vi "Teleop.vi"(10 "Match Info":T1={"Autonomous Elapsed Seconds"=0.0, "TeleOp Elapsed Seconds"=0.0, "Disabled Elapsed Seconds"=0.0, "Visited Autonomous"=FALSE, "Visited TeleOp"=FALSE, "Visited Disabled"=FALSE, "Autonomous Settings"={"Autonomous Style"=enum."Independent", "VI Refnum"=refnum}}, 11 "Call Context":T2) -> ()   [LabVIEW 2014]
doc: "This VI is called for each TeleOp packet received from the DS where the robot is not disabled. It is often used to read from the joysticks and update I/O or to update setpoints for timed control loops. It should complete and return within 20 milliseconds or it may miss DS packets."
uses:
  <vilib>/Rock Robotics/WPI/DriverStation/WPI_DriverStationDerivedRobotMode.ctl
  <vilib>/Rock Robotics/WPI/DriverStation/WPI_DriverStationMatch Info.ctl
  <vilib>/Rock Robotics/Network Tables/SD Read Boolean.vi
  <vilib>/Rock Robotics/Network Tables/SD Read Number.vi
  <vilib>/Rock Robotics/WPI/RobotDrive/WPI_RobotDriveGetSetRefNum.vi
  <vilib>/Rock Robotics/WPI/Joystick/WPI_JoystickGetSetRefNum.vi
  <vilib>/Rock Robotics/Network Tables/SD Write Numeric Array.vi
  <vilib>/Rock Robotics/Network Tables/SD Write Boolean Array.vi
  <vilib>/Rock Robotics/WPI/RobotDrive/WPI_RobotDriveMecanumDrive_Cartesian.vi
  Robot Global Data.vi
  <vilib>/addons/control/pid/NI_PID_pid.lvlib
  <vilib>/addons/control/pid/pid.llb/PID (DBL).vi
panel:
  out "Sample Slider 0":dbl(slide) scale=0.0..5.0
  out "Sample Boolean 1":bool
  out "Sample Boolean 0":bool
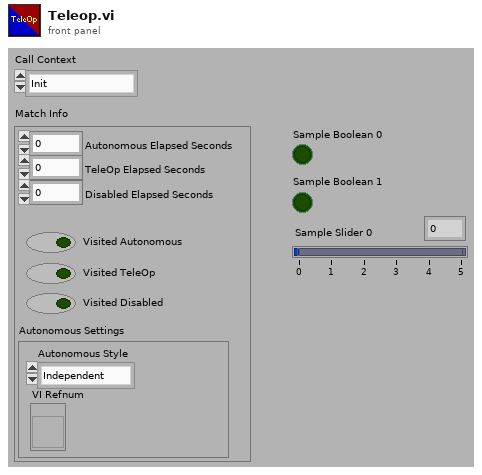
[diagram p1: front panel]
types:
  T1 = typedef "WPI_DriverStationMatch Info.ctl" = cluster{"Autonomous Elapsed Seconds":dbl, "TeleOp Elapsed Seconds":dbl, "Disabled Elapsed Seconds":dbl, "Visited Autonomous":bool, "Visited TeleOp":bool, "Visited Disabled":bool, "Autonomous Settings":cluster{"Autonomous Style":enum16{"Iterative", "Independent"}, "VI Refnum":refnum<vi>}}
  T2 = typedef "WPI_DriverStationDerivedRobotMode.ctl" = enum16{"Init", "Execute", "Stop"}
  T3 = enum16{"straight", "L1", "L2", "R1", "R2", "trigger"}
  T4 = typedef "WPI_JoystickDevRef.ctl" = cluster{"Device":T5}
  T5 = typedef "WPI_JoystickDeviceEnum.ctl" = enum16{"USB 0", "USB 1", "USB 2", "USB 3", "USB 4", "USB 5"}
  T6 = typedef "WPI_GyroDevRef.ctl" = cluster{"DevStatus":errorcluster, "Analog Module":T7, "Analog Channel":T8, "Offset":dbl, "Gain (VoltsPerDegree/Second)":dbl}
  T7 = typedef "FPGA_TypedefAnalogModule.ctl" = enum16{"Controller 1"}
  T8 = typedef "FPGA_AIChannel.ctl" = enum8{"AI 0", "AI 1", "AI 2", "AI 3", "AI MXP 0", "AI MXP 1", "AI MXP 2", "AI MXP 3", "Invalid"}
  T9 = typedef "WPI_RobotDriveDevRef.ctl" = cluster{"DevStatus":errorcluster, "Motors[]":T10[], "Square Inputs":bool, "Max Output":dbl}
  T10 = typedef "WPI_MotorControlDeviceRef.ctl" = cluster{"DeviceStatus":errorcluster, "Type":T11, "PWM":cluster{"Controller":T12, "PWM Channel":T13, "DeadBand":T14}, "CAN":cluster{"Device Number":u8, "Control Mode":T15, "Semaphore":T16, "Max Vout":dbl, "TalonSRX Control Mode":T17}, "Invert":bool, "TransformRef":T18, "InvTransformRef":T18}
  T11 = typedef "WPI_MotorControlType.ctl" = enum16{"PWM", "CAN", "CANTalonSRX"}
  T12 = typedef "FPGA_TypedefDigitalModule.ctl" = enum16{"Controller 1"}
  T13 = typedef "FPGA_DIOPWMChannel.ctl" = enum8{"PWM 0", "PWM 1", "PWM 2", "PWM 3", "PWM 4", "PWM 5", "PWM 6", "PWM 7", "PWM 8", "PWM 9", "PWM MXP 0", "PWM MXP 1", "PWM MXP 2", "PWM MXP 3", "PWM MXP 4", "PWM MXP 5", "PWM MXP 6", "PWM MXP 7", "PWM MXP 8", "PWM MXP 9", "Invalid"}
  T14 = typedef "WPI_PWMDeadband.ctl" = cluster{"Name":string, "maxPositivePwm":i32, "minPositivePwm":i32, "centerPwm":i32, "maxNegativePwm":i32, "minNegativePwm":i32, "angularRange":u16}
  T15 = typedef "WPI_CANJaguar_ControlMode.ctl" = enum8{"Percent VBus", "Current", "Speed", "Position", "Voltage"}
  T16 = typedef "Semaphore RefNum" = refnum<k1>
  T17 = typedef "WPI_CANTalonSRX_APIControlMode.ctl" = enum8{"Percent VBus", "Speed", "Position", "Slave", "Unchanged / Invalid"}
  T18 = typedef "WPI_PWMTransform_ConPane.ctl" = refnum<vi>
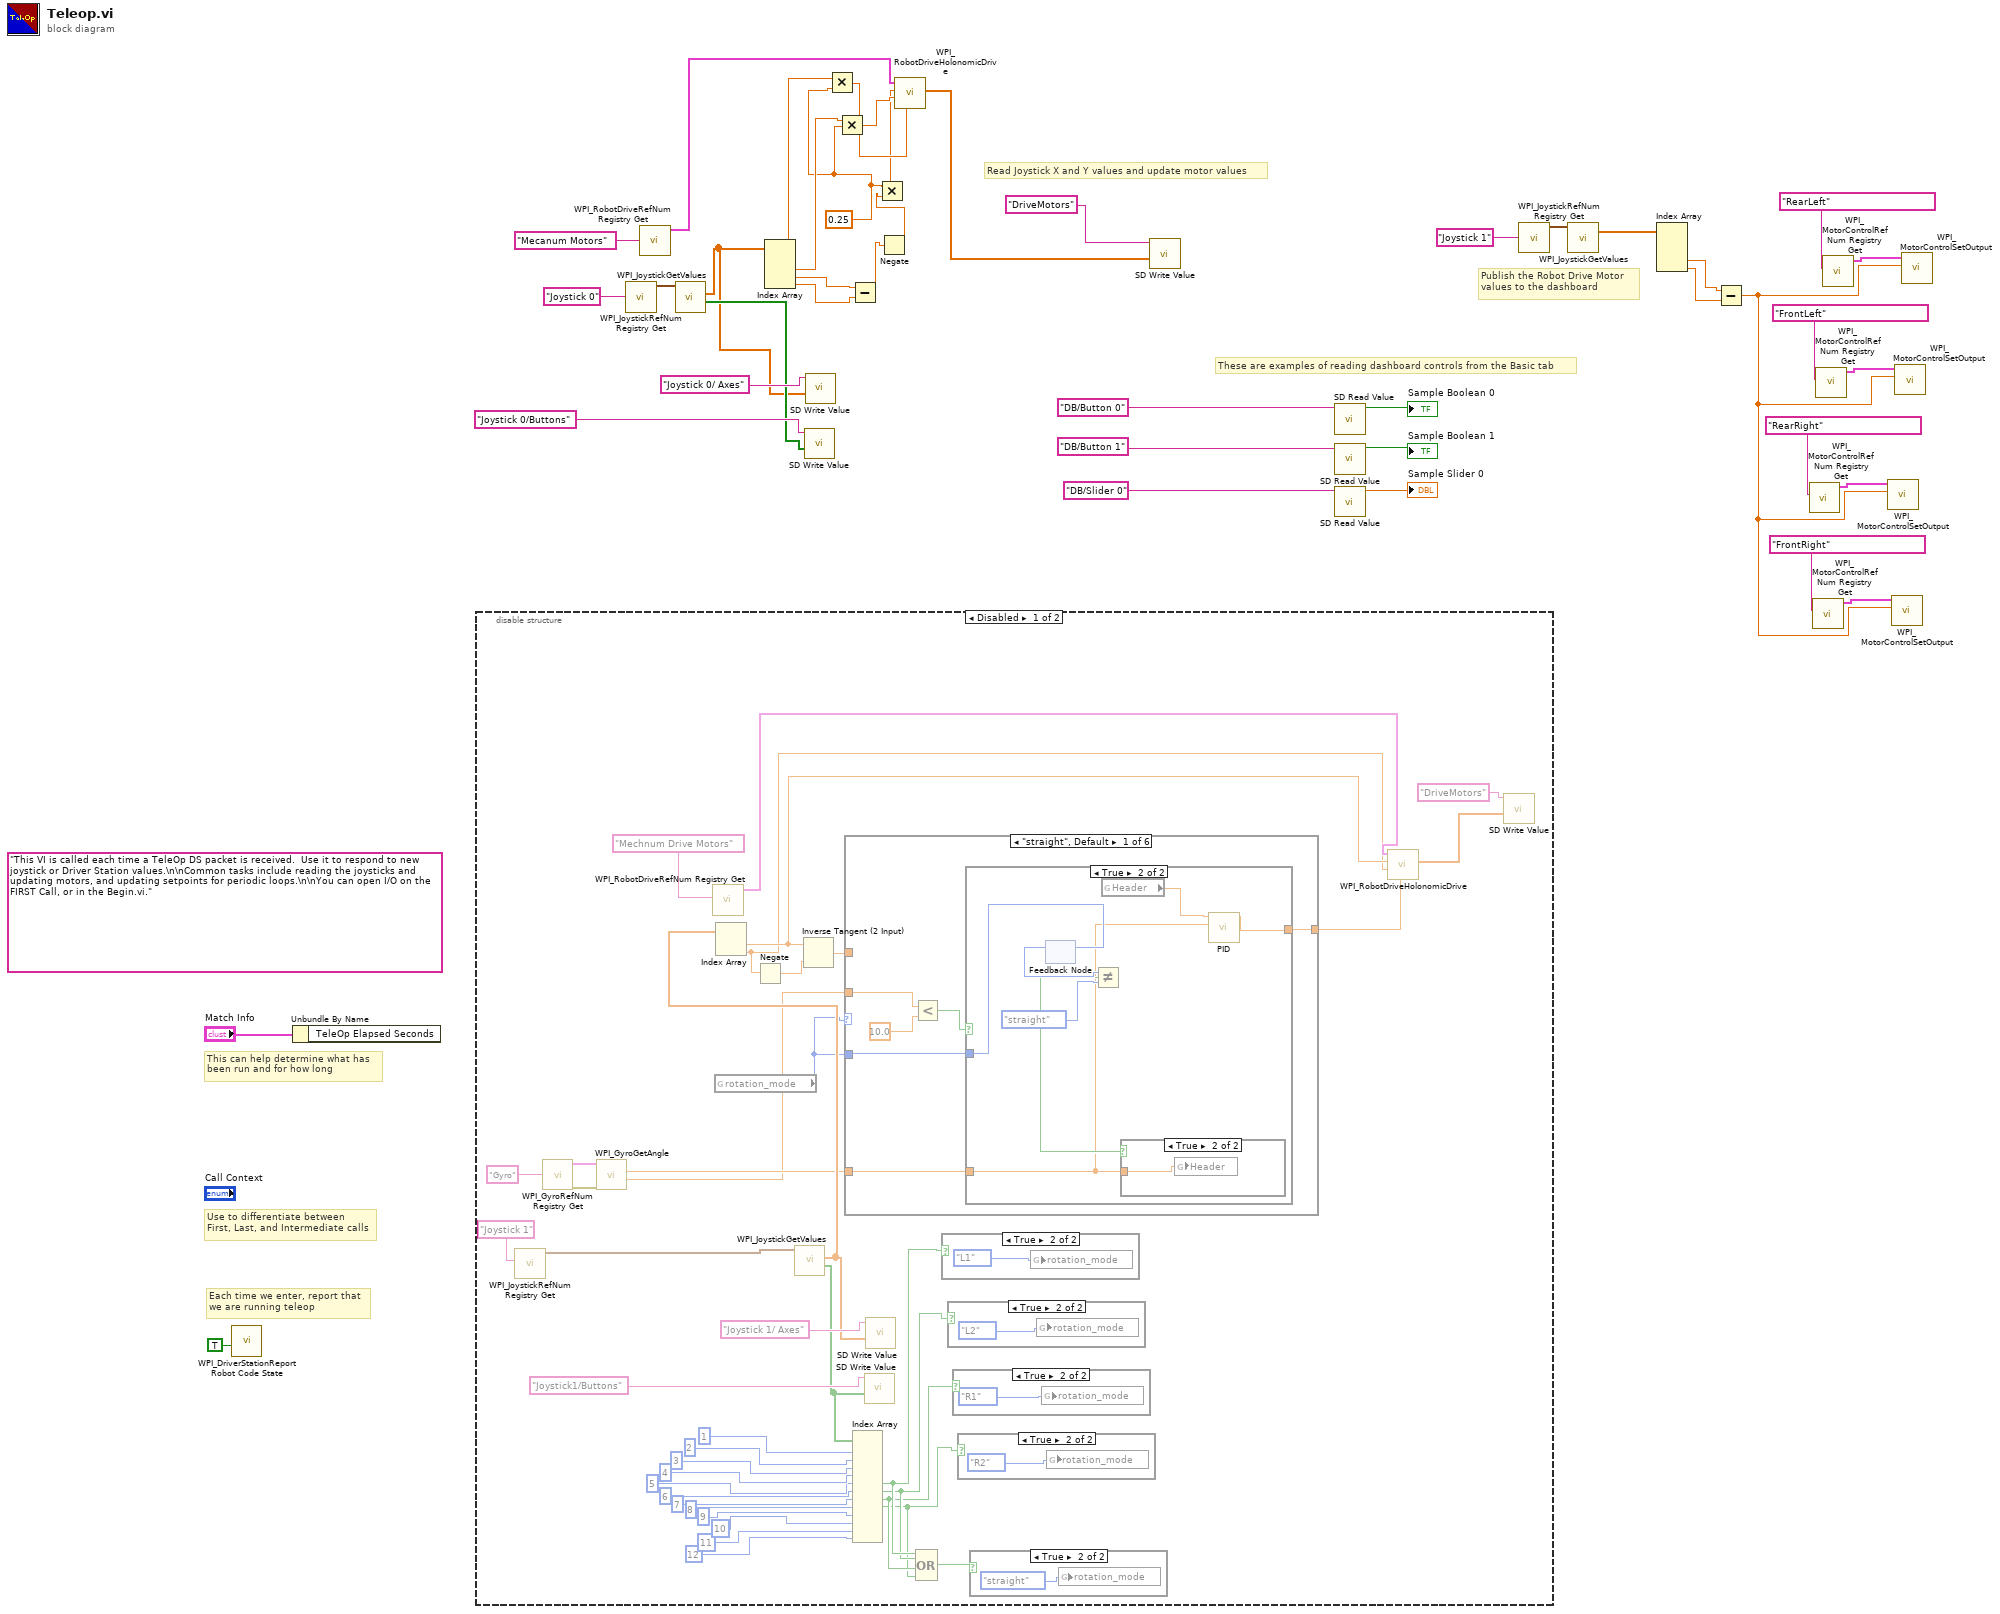
[diagram p0: block diagram]
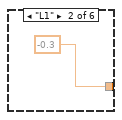
[diagram p9: hidden frame]
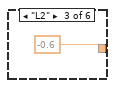
[diagram p10: hidden frame]
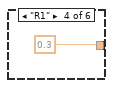
[diagram p11: hidden frame]
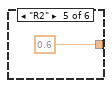
[diagram p12: hidden frame]
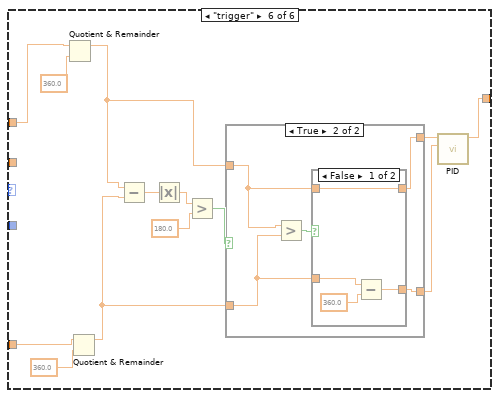
[diagram p13: hidden frame]
diagram:
  w3 = 0.25
  (unwired) "This VI is called each time a TeleOp DS packet is received.  Use it to respond to new joystick or Driver Station values.\n\nCommon tasks include reading the joysticks and updating motors, and updating setpoints for periodic loops.\n\nYou can open I/O on the FIRST Call, or in the Begin.vi."
  # "Publish the Robot Drive Motor\nvalues to the dashboard"
  # "Read Joystick X and Y values and update motor values"
  # "These are examples of reading dashboard controls from the Basic tab"
  # "Each time we enter, report that\nwe are running teleop"
  # "Use to differentiate between\nFirst, Last, and Intermediate calls"
  # "This can help determine what has\nbeen run and for how long"
  n1 = call <vilib>:"WPI_DriverStationReport Robot Code State.vi"("TeleOp"=TRUE ("Autonomous")) -> ()  [unwired: 10 in, 1 out]
  n2 = Unbundle By Name("Match Info") -> ()  [unwired: 1 out]
  n3 = disable-structure shown="Disabled" {
    frame Disabled {
      n4 = call <vilib>:"WPI_JoystickRefNum Registry Get.vi"("refnum name"="Joystick 1") -> ("JoystickDevRef"=w75:T4)  [unwired: 1 in, 9 out]
      n5 = call <vilib>:"WPI_GyroRefNum Registry Get.vi"("refnum name"="Gyro") -> ("error out"=w65:errorcluster, "GyroDevRef"=w64:T6)  [unwired: 9 in]
      n6 = call <vilib>:"WPI_GyroGetAngle.vi"("error in (no error)"=w65, "GyroDevRef"=w64) -> ("Angular Rate"=w43:dbl, "Angle"=w44:dbl)  [unwired: 6 in, 2 out]
      n7 = call <vilib>:"WPI_RobotDriveRefNum Registry Get.vi"("refnum name"="Mechnum Drive Motors") -> ("RobotDriveDevRef"=w70:T9)  [unwired: 1 in, 9 out]
      n8 = global read "Robot Global Data.vi" "rotation_mode"() -> (w51:T3)
      n9 = call <vilib>:"WPI_JoystickGetValues.vi"("JoystickDevRef"=w75) -> ("Buttons"=w74:bool[], "Axes"=w72:dbl[])  [unwired: 6 in, 3 out]
      n10 = Index Array(array=w72) -> (element #1=w71:dbl, element #2=w69:dbl)  [unwired: 2 in]
      n11 = Negate(x=w69) -> (-x=w68:dbl)
      n12 = Inverse Tangent (2 Input)(1:w68, 2:w71) -> (0:w67:dbl)
      n13 = case shown="\"straight\", Default" w51 {
        tunnel: w67 -> [_ _ _ _ _ w116]
        tunnel: w51 -> [w91 _ _ _ _ _]
        tunnel: [w86 -0.3 -0.6 0.3 0.6 w107] -> w50
        tunnel: w44 -> [w90 _ _ _ _ w114]
        tunnel: w43 -> [w87 _ _ _ _ _]
        frame "straight", Default {
          n14 = Less?(x=w87, y=10.0) -> (x < y?=w89:bool)
          n15 = case shown="True" w89 {
            tunnel: [w92 w95] -> w86
            tunnel: w91 -> [_ w94]
            tunnel: w90 -> [w92 w93]
            frame False {
            }
            frame True {
              n16 = feedback #1() -> (w99:T3)  [unwired: 1 in]
              n17 = feedback-in #1(w94) -> ()
              n18 = Not Equal?(x=w99, y=T3."straight") -> (x != y?=w97:bool)
              n19 = global read "Robot Global Data.vi" "Header"() -> (w96:dbl)
              n20 = case shown="True" w97 {
                tunnel: w93 -> [_ w100]
                frame False {
                }
                frame True {
                  n21 = global write "Robot Global Data.vi" "Header"(w100) -> ()
                }
              }
              n22 = call-poly <vilib>:"PID.vi"("process variable"=w93, "setpoint"=w96) -> ("output"=w95:dbl)  [unwired: 8 in, 1 out]
            }
          }
        }
        frame "L1" {
        }
        frame "L2" {
        }
        frame "R1" {
        }
        frame "R2" {
        }
        frame "trigger" {
          n23 = Quotient & Remainder(x=w116, y=360.0) -> (x-y*floor(x/y)=w109:dbl)  [unwired: 1 out]
          n24 = Quotient & Remainder(x=w114, y=360.0) -> (x-y*floor(x/y)=w108:dbl)  [unwired: 1 out]
          n25 = Subtract(x=w109, y=w108) -> (x-y=w113:dbl)
          n26 = Absolute Value(x=w113) -> (abs(x)=w112:dbl)
          n27 = Greater?(x=w112, y=180.0) -> (0:w110:bool)
          n28 = case shown="True" w110 {
            tunnel: w109 -> [w118 w123]
            tunnel: w108 -> [w119 w122]
            tunnel: [w119 w120] -> w106
            tunnel: [w118 w121] -> w105
            frame False {
            }
            frame True {
              n29 = Greater?(x=w123, y=w122) -> (0:w124:bool)
              n30 = case shown="False" w124 {
                tunnel: w123 -> [w127 w130]
                tunnel: w122 -> [w126 w129]
                tunnel: [w127 w130] -> w121
                tunnel: [w125 w129] -> w120
                frame False {
                  n31 = Subtract(x=w126, y=360.0) -> (x-y=w125:dbl)
                }
                frame True {
                }
              }
            }
          }
          n32 = call-poly <vilib>:"PID.vi"("process variable"=w106, "setpoint"=w105) -> ("output"=w107:dbl)  [unwired: 8 in, 1 out]
        }
      }
      n33 = Index Array(array=w74, index #1=1, index #2=2, index #3=3, index #4=4, index #5=5, index #6=6, index #7=7, index #8=8, index #9=9, index #10=10, index #11=11, index #12=12) -> (element #5=w49:bool, element #6=w48:bool, element #7=w47:bool, element #8=w46:bool)  [unwired: 8 out]
      n34 = call-poly <vilib>:"SD Write Value.vi"("Boolean Array"=w74, "Name"="Joystick1/Buttons") -> ()  [unwired: 8 in, 2 out]
      n35 = call-poly <vilib>:"SD Write Value.vi"("Numeric Array"=w72, "Name"="Joystick 1/ Axes") -> ()  [unwired: 8 in, 2 out]
      n36 = Compound Arithmetic op=OR(w49, w48, w47, w46) -> (w45:bool)
      n37 = case shown="True" w49 {
        frame False {
        }
        frame True {
          n38 = global write "Robot Global Data.vi" "rotation_mode"(T3."L1") -> ()
        }
      }
      n39 = case shown="True" w48 {
        frame False {
        }
        frame True {
          n40 = global write "Robot Global Data.vi" "rotation_mode"(T3."L2") -> ()
        }
      }
      n41 = case shown="True" w47 {
        frame False {
        }
        frame True {
          n42 = global write "Robot Global Data.vi" "rotation_mode"(T3."R1") -> ()
        }
      }
      n43 = case shown="True" w46 {
        frame False {
        }
        frame True {
          n44 = global write "Robot Global Data.vi" "rotation_mode"(T3."R2") -> ()
        }
      }
      n45 = case shown="True" w45 {
        frame False {
        }
        frame True {
          n46 = global write "Robot Global Data.vi" "rotation_mode"(T3."straight") -> ()
        }
      }
      n47 = call-poly <vilib>:"WPI_RobotDriveHolonomicDrive.vi"("Rotation"=w50, "Y"=w69, "X"=w71, "RobotDriveDevRef"=w70) -> ("Motor Values"=w77:dbl[])  [unwired: 5 in, 2 out]
      n48 = call-poly <vilib>:"SD Write Value.vi"("Numeric Array"=w77, "Name"="DriveMotors") -> ()  [unwired: 8 in, 2 out]
    }
    frame Enabled {
    }
  }
  n49 = call <vilib>:"WPI_JoystickRefNum Registry Get.vi"("refnum name"="Joystick 0") -> ("JoystickDevRef"=w23:T4)  [unwired: 9 in, 1 out]
  n50 = call <vilib>:"WPI_RobotDriveRefNum Registry Get.vi"("refnum name"="Mecanum Motors") -> ("RobotDriveDevRef"=w14:T9)  [unwired: 9 in, 1 out]
  n51 = call <vilib>:"WPI_JoystickGetValues.vi"("JoystickDevRef"=w23) -> ("Buttons"=w20:bool[], "Axes"=w19:dbl[])  [unwired: 6 in, 3 out]
  n52 = Index Array(array=w19) -> (element #1=w13:dbl, element #2=w12:dbl, element #3=w6:dbl, element #4=w5:dbl)  [unwired: 4 in]
  n53 = call-poly <vilib>:"SD Write Value.vi"("Boolean Array"=w20, "Name"="Joystick 0/Buttons") -> ()  [unwired: 8 in, 2 out]
  n54 = call-poly <vilib>:"SD Write Value.vi"("Numeric Array"=w19, "Name"="Joystick 0/ Axes") -> ()  [unwired: 8 in, 2 out]
  n55 = Multiply(x=w13, y=w3) -> (x*y=w7:dbl)
  n56 = Multiply(x=w12, y=w3) -> (x*y=w11:dbl)
  n57 = Subtract(x=w6, y=w5) -> (x-y=w4:dbl)
  n58 = Negate(x=w4) -> (-x=w2:dbl)
  n59 = Multiply(x=w3, y=w2) -> (x*y=w1:dbl)
  n60 = call-poly <vilib>:"WPI_RobotDriveHolonomicDrive.vi"("Rotation"=w7, "Y"=w11, "X"=w1, "RobotDriveDevRef"=w14) -> ("Motor Values"=w18:dbl[])  [unwired: 5 in, 2 out]
  n61 = call-poly <vilib>:"SD Write Value.vi"("Numeric Array"=w18, "Name"="DriveMotors") -> ()  [unwired: 8 in, 2 out]
  n62 = call-poly <vilib>:"SD Read Value.vi"("Name"="DB/Button 0" ("refnum name")) -> ("Boolean"=→"Sample Boolean 0":bool)  [unwired: 8 in, 2 out]
  n63 = call-poly <vilib>:"SD Read Value.vi"("Name"="DB/Button 1" ("refnum name")) -> ("Boolean"=→"Sample Boolean 1":bool)  [unwired: 8 in, 2 out]
  n64 = call-poly <vilib>:"SD Read Value.vi"("Name"="DB/Slider 0" ("refnum name")) -> ("Numeric"=→"Sample Slider 0":dbl)  [unwired: 8 in, 2 out]
  n65 = call <vilib>:"WPI_JoystickRefNum Registry Get.vi"("refnum name"="Joystick 1") -> ("JoystickDevRef"=w15:T4)  [unwired: 9 in, 1 out]
  n66 = call <vilib>:"WPI_JoystickGetValues.vi"("JoystickDevRef"=w15) -> ("Axes"=w10:dbl[])  [unwired: 6 in, 4 out]
  n67 = Index Array(array=w10) -> (element #3=w9:dbl, element #4=w8:dbl)  [unwired: 4 in, 2 out]
  n68 = Subtract(x=w9, y=w8) -> (x-y=w26:dbl)
  n69 = call <vilib>:"WPI_MotorControlRefNum Registry Get.vi"("refnum name"="RearRight") -> ("MotorControlDevRef"=w28:T10)  [unwired: 9 in, 1 out]
  n70 = call <vilib>:"WPI_MotorControlRefNum Registry Get.vi"("refnum name"="FrontRight") -> ("MotorControlDevRef"=w31:T10)  [unwired: 9 in, 1 out]
  n71 = call <vilib>:"WPI_MotorControlRefNum Registry Get.vi"("refnum name"="FrontLeft") -> ("MotorControlDevRef"=w30:T10)  [unwired: 9 in, 1 out]
  n72 = call <vilib>:"WPI_MotorControlRefNum Registry Get.vi"("refnum name"="RearLeft") -> ("MotorControlDevRef"=w34:T10)  [unwired: 9 in, 1 out]
  n73 = call <vilib>:"WPI_MotorControlSetOutput.vi"("Output"=w26, "MotorControlDevRef"=w28) -> ()  [unwired: 7 in, 3 out]
  n74 = call <vilib>:"WPI_MotorControlSetOutput.vi"("Output"=w26, "MotorControlDevRef"=w31) -> ()  [unwired: 7 in, 3 out]
  n75 = call <vilib>:"WPI_MotorControlSetOutput.vi"("Output"=w26, "MotorControlDevRef"=w30) -> ()  [unwired: 7 in, 3 out]
  n76 = call <vilib>:"WPI_MotorControlSetOutput.vi"("Output"=w26, "MotorControlDevRef"=w34) -> ()  [unwired: 7 in, 3 out]
